vi "Build Assert Variant.vi"(8 "error in (no error)":errorcluster, 10 "Assert Data":T1, 11 "Assert Variant in":variant) -> (0 "error out":errorcluster, 3 "Assert Variant out":variant)   [LabVIEW 2016, in "AssertEngine.lvlib" / "AssertEngine.lvclass"]
doc: "Builds up an assert configuration based on the Assert Data provided"
uses:
  AssertEngine.lvclass
  Log Assert/Assert Data.ctl
  Private Constants.vi
  <vilib>/Utility/Data Type/NI_Data Type.lvlib
  AssertEngine.lvlib
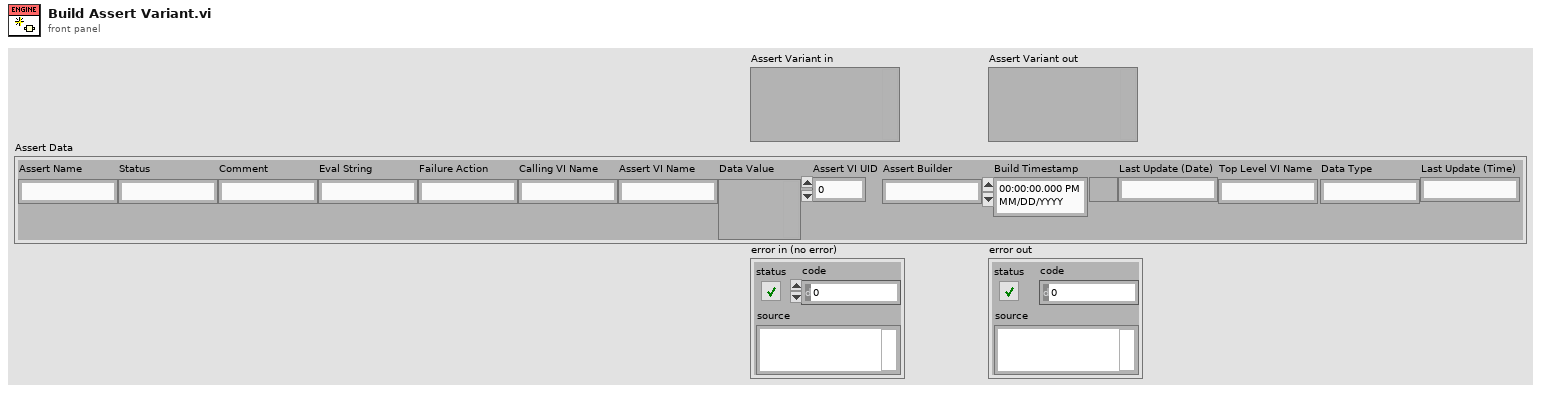
[diagram p1: front panel]
types:
  T1 = typedef "AssertEngine.lvlib/Assert Data.ctl" = cluster{"Assert Name":string, "Status":string, "Comment":string, "Eval String":string, "Failure Action":string, "Calling VI Name":string, "Assert VI Name":string, "Data Value":variant, "Assert VI UID":i32, "Assert Builder":string, "Build Timestamp":timestamp, "Last Update (Date)":string, "Top Level VI Name":string, "Data Type":string, "Last Update (Time)":string}
  T2 = typedef "NI_Data Type.lvlib/Data Type.ctl" = enum8{"Invalid Type", "Void", "I8", "I16", "I32", "I64", "U8", "U16", "U32", "U64", "Single Float", "Double Float", "Extended Float", "Single Complex", "Double Complex", "Extended Complex", "Enum U8", "Enum U16", "Enum U32", "Enum U64", "Single Float With Unit", "Double Float With Unit", "Extended Float With Unit", "Single Complex with Unit", "Double Complex with Unit", "Extended Complex with Unit", "Boolean", "String", "Path", "Picture", "Tag", "Array", "Cluster", "Variant", "LV Variant", "Waveform", "Timestamp", "Digital Waveform", "Digital Data", "ExpressData", "Refnum", "External Data", "VI", "Poly VI", "LabVIEW Class Instance", "Fixed Point"}
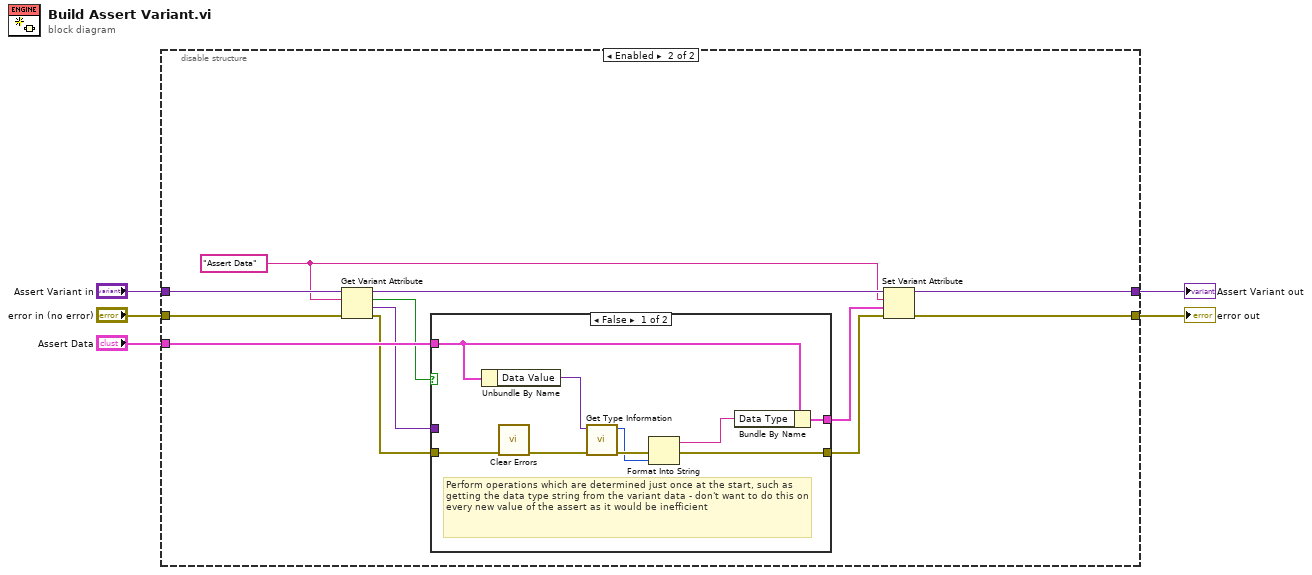
[diagram p0: block diagram]
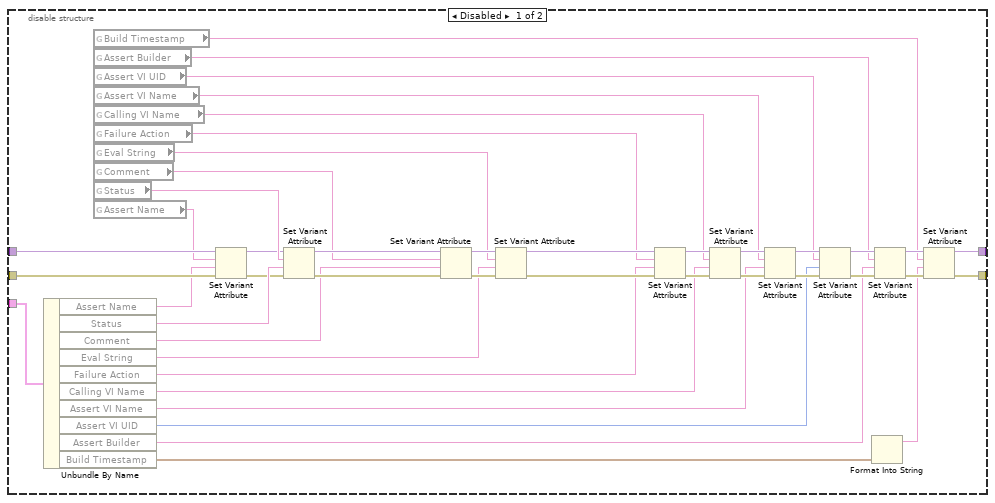
[diagram p2: hidden frame]
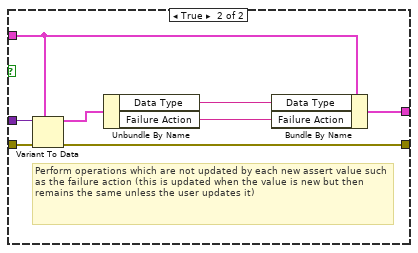
[diagram p3: hidden frame]
diagram:
  n1 = disable-structure shown="Enabled" {
    disable-tunnel: "Assert Data" -> [w47 w55]
    disable-tunnel: "error in (no error)" -> [w45 w61]
    disable-tunnel: "Assert Variant in" -> [w31 w58]
    disable-tunnel: [w11 w60] -> w2
    disable-tunnel: [w9 w59] -> w1
    frame Disabled {
      n2 = Unbundle By Name(w47) -> ("Assert Name"=w28:string, "Status"=w48:string, "Comment"=w27:string, "Eval String"=w26:string, "Failure Action"=w25:string, "Calling VI Name"=w24:string, "Assert VI Name"=w23:string, "Assert VI UID"=w22:i32, "Assert Builder"=w13:string, "Build Timestamp"=w7:timestamp)
      n3 = global read "Private Constants.vi" "Build Timestamp"() -> (w8:string)
      n4 = global read "Private Constants.vi" "Assert Builder"() -> (w12:string)
      n5 = global read "Private Constants.vi" "Assert VI UID"() -> (w14:string)
      n6 = global read "Private Constants.vi" "Assert VI Name"() -> (w15:string)
      n7 = global read "Private Constants.vi" "Calling VI Name"() -> (w16:string)
      n8 = global read "Private Constants.vi" "Failure Action"() -> (w17:string)
      n9 = global read "Private Constants.vi" "Eval String"() -> (w18:string)
      n10 = global read "Private Constants.vi" "Comment"() -> (w19:string)
      n11 = global read "Private Constants.vi" "Status"() -> (w49:string)
      n12 = global read "Private Constants.vi" "Assert Name"() -> (w29:string)
      n13 = Set Variant Attribute(Variant=w31, name=w29, value=w28, error in=w45) -> (Variant out=w30:variant, error out=w32:errorcluster)  [unwired: 1 out]
      n14 = Set Variant Attribute(Variant=w30, name=w49, value=w48, error in=w32) -> (Variant out=w41:variant, error out=w46:errorcluster)  [unwired: 1 out]
      n15 = Set Variant Attribute(Variant=w41, name=w19, value=w27, error in=w46) -> (Variant out=w40:variant, error out=w42:errorcluster)  [unwired: 1 out]
      n16 = Set Variant Attribute(Variant=w40, name=w18, value=w26, error in=w42) -> (Variant out=w38:variant, error out=w43:errorcluster)  [unwired: 1 out]
      n17 = Set Variant Attribute(Variant=w38, name=w17, value=w25, error in=w43) -> (Variant out=w37:variant, error out=w39:errorcluster)  [unwired: 1 out]
      n18 = Set Variant Attribute(Variant=w37, name=w16, value=w24, error in=w39) -> (Variant out=w34:variant, error out=w44:errorcluster)  [unwired: 1 out]
      n19 = Set Variant Attribute(Variant=w34, name=w15, value=w23, error in=w44) -> (Variant out=w33:variant, error out=w35:errorcluster)  [unwired: 1 out]
      n20 = Set Variant Attribute(Variant=w33, name=w14, value=w22, error in=w35) -> (Variant out=w20:variant, error out=w36:errorcluster)  [unwired: 1 out]
      n21 = Format Into String(w7) -> (resulting string=w6:string)  [unwired: 3 in, 1 out]
      n22 = Set Variant Attribute(Variant=w20, name=w12, value=w13, error in=w36) -> (Variant out=w10:variant, error out=w21:errorcluster)  [unwired: 1 out]
      n23 = Set Variant Attribute(Variant=w10, name=w8, value=w6, error in=w21) -> (Variant out=w9:variant, error out=w11:errorcluster)  [unwired: 1 out]
    }
    frame Enabled {
      w56 = "Assert Data"
      n24 = Get Variant Attribute(Variant=w58, name=w56, error in=w61) -> (duplicate Variant=w57:variant, found=w51:bool, value=w54:variant, error out=w53:errorcluster)  [unwired: 1 in]
      n25 = case shown="False" w51 {
        tunnel: w55 -> [w68 w78]
        tunnel: w54 -> [_ w77]
        tunnel: w53 -> [w70 w76]
        tunnel: [w63 w75] -> w52
        tunnel: [w65 w72] -> w50
        frame False {
          # "Perform operations which are determined just once at the start, such as getting the data type string from the variant data - don't want to do this on every new value of the assert as it would be inefficient"
          n26 = Unbundle By Name(w68) -> ("Data Value"=w66:variant)
          n27 = call <vilib>:"Clear Errors.vi"("error in (no error)"=w70) -> ("error out"=w69:errorcluster)  [unwired: 5 in, 1 out]
          n28 = call <vilib>:"Get Type Information.vi"("error in (no error)"=w69, "Variant"=w66) -> ("error out"=w67:errorcluster, "Type"=w64:T2)  [unwired: 5 in, 3 out]
          n29 = Format Into String(error in=w67, w64) -> (resulting string=w62:string, error out=w65:errorcluster)  [unwired: 2 in]
          n30 = Bundle By Name(cluster=w68, "Data Type"=w62) -> (w63:T1)
        }
        frame True {
          # "Perform operations which are not updated by each new assert value such as the failure action (this is updated when the value is new but then remains the same unless the user updates it)"
          n31 = Variant To Data(error in=w76, type=w78, Variant=w77) -> (data=w74:T1, error out=w72:errorcluster)
          n32 = Unbundle By Name(w74) -> ("Data Type"=w71:string, "Failure Action"=w73:string)
          n33 = Bundle By Name(cluster=w78, "Data Type"=w71, "Failure Action"=w73) -> (w75:T1)
        }
      }
      n34 = Set Variant Attribute(Variant=w57, name=w56, value=w52, error in=w50) -> (Variant out=w59:variant, error out=w60:errorcluster)  [unwired: 1 out]
    }
  }
  "error out" <- w2
  "Assert Variant out" <- w1
